vi "Serial_Check.vi"() -> ()   [LabVIEW 2014]
uses:
  <vilib>/Instr/_visa.llb/VISA Configure Serial Port (Instr).vi
  user32.dll
panel:
  in  "정지":bool
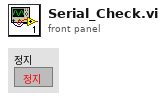
[diagram p1: front panel]
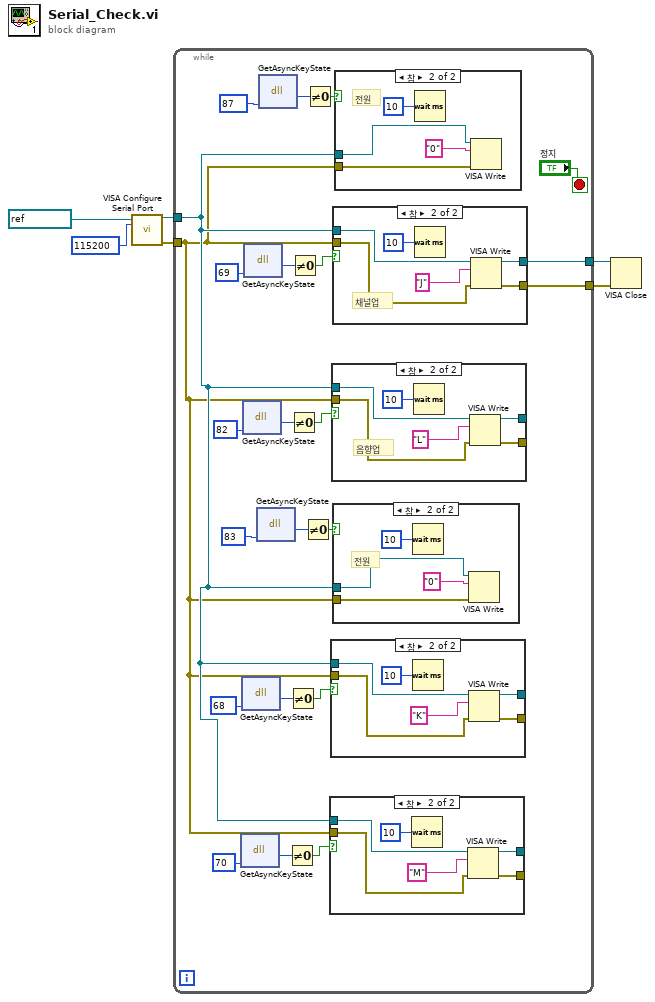
[diagram p0: block diagram]
diagram:
  n1 = call-poly "VISA Configure Serial Port"("VISA resource name"=refnum<visa-resource-name> "COM3", "baud rate (9600)"=u32 115200) -> ("VISA resource name out"=w4:refnum<visa-resource-name>, "error out"=w5:errorcluster)  [unwired: 12 in]
  n2 = while {
    tunnel: w5 -> [w7]
    tunnel: w4 -> [w8]
    tunnel: [w28] -> w3
    tunnel: [w27] -> w2
    stop <- "정지" stop-if-true
    n3 = dll-call lib="User32.dll" fn="GetAsyncKeyState"("vKey"=u8 70 ("Receive_Interaction")) -> ("return type"=w17:i64)  [unwired: 4 in, 2 out]
    n4 = dll-call lib="User32.dll" fn="GetAsyncKeyState"("vKey"=u8 68 ("Receive_Interaction")) -> ("return type"=w12:i64)  [unwired: 4 in, 2 out]
    n5 = dll-call lib="User32.dll" fn="GetAsyncKeyState"("vKey"=u8 82 ("Receive_Interaction")) -> ("return type"=w18:i64)  [unwired: 4 in, 2 out]
    n6 = dll-call lib="User32.dll" fn="GetAsyncKeyState"("vKey"=u8 69 ("Receive_Interaction")) -> ("return type"=w23:i64)  [unwired: 4 in, 2 out]
    n7 = dll-call lib="User32.dll" fn="GetAsyncKeyState"("vKey"=u8 83 ("Receive_Interaction")) -> ("return type"=w10:i64)  [unwired: 4 in, 2 out]
    n8 = dll-call lib="User32.dll" fn="GetAsyncKeyState"("vKey"=u8 87 ("Receive_Interaction")) -> ("return type"=w25:i64)  [unwired: 4 in, 2 out]
    n9 = Not Equal To 0?(x=w17) -> (x != 0?=w15:bool)
    n10 = Not Equal To 0?(x=w12) -> (x != 0?=w14:bool)
    n11 = Not Equal To 0?(x=w18) -> (x != 0?=w20:bool)
    n12 = Not Equal To 0?(x=w23) -> (x != 0?=w21:bool)
    n13 = Not Equal To 0?(x=w10) -> (x != 0?=w11:bool)
    n14 = Not Equal To 0?(x=w25) -> (x != 0?=w24:bool)
    n15 = case shown="참" w15 {
      tunnel: w7 -> [w30 w36]
      tunnel: w8 -> [w31 w35]
      tunnel: [w31 w34] -> _
      tunnel: [w30 w33] -> _
      frame False {
      }
      frame True {
        n16 = Wait (ms)(milliseconds to wait=u32 10 ("대기 시간(ms)")) -> ()  [unwired: 1 out]
        n17 = VISA Write(VISA resource name=w35, write buffer="M", error in (no error)=w36) -> (VISA resource name out=w34:refnum<visa-resource-name>, error out=w33:errorcluster)  [unwired: 1 out]
      }
    }
    n18 = case shown="참" w14 {
      tunnel: w7 -> [w42 w48]
      tunnel: w8 -> [w43 w47]
      tunnel: [w43 w46] -> _
      tunnel: [w42 w45] -> _
      frame False {
      }
      frame True {
        n19 = Wait (ms)(milliseconds to wait=u32 10 ("대기 시간(ms)")) -> ()  [unwired: 1 out]
        n20 = VISA Write(VISA resource name=w47, write buffer="K", error in (no error)=w48) -> (VISA resource name out=w46:refnum<visa-resource-name>, error out=w45:errorcluster)  [unwired: 1 out]
      }
    }
    n21 = case shown="참" w20 {
      tunnel: w7 -> [w50 w56]
      tunnel: w8 -> [w51 w55]
      tunnel: [w51 w54] -> _
      tunnel: [w50 w53] -> _
      frame False {
      }
      frame True {
        # "음향업"
        n22 = Wait (ms)(milliseconds to wait=u32 10 ("대기 시간(ms)")) -> ()  [unwired: 1 out]
        n23 = VISA Write(VISA resource name=w55, write buffer="L", error in (no error)=w56) -> (VISA resource name out=w54:refnum<visa-resource-name>, error out=w53:errorcluster)  [unwired: 1 out]
      }
    }
    n24 = case shown="참" w21 {
      tunnel: w7 -> [w62 w68]
      tunnel: w8 -> [w63 w67]
      tunnel: [w63 w66] -> w28
      tunnel: [w62 w65] -> w27
      frame False {
      }
      frame True {
        # "채널업"
        n25 = Wait (ms)(milliseconds to wait=u32 10 ("대기 시간(ms)")) -> ()  [unwired: 1 out]
        n26 = VISA Write(VISA resource name=w67, write buffer="J", error in (no error)=w68) -> (VISA resource name out=w66:refnum<visa-resource-name>, error out=w65:errorcluster)  [unwired: 1 out]
      }
    }
    n27 = case shown="참" w11 {
      tunnel: w7 -> [_ w40]
      tunnel: w8 -> [_ w39]
      frame False {
      }
      frame True {
        # "전원"
        n28 = Wait (ms)(milliseconds to wait=u32 10 ("대기 시간(ms)")) -> ()  [unwired: 1 out]
        n29 = VISA Write(VISA resource name=w39, write buffer="0" ("write buffer 2"), error in (no error)=w40) -> ()  [unwired: 3 out]
      }
    }
    n30 = case shown="참" w24 {
      tunnel: w7 -> [_ w60]
      tunnel: w8 -> [_ w59]
      frame False {
      }
      frame True {
        # "전원"
        n31 = Wait (ms)(milliseconds to wait=u32 10 ("대기 시간(ms)")) -> ()  [unwired: 1 out]
        n32 = VISA Write(VISA resource name=w59, write buffer="0" ("write buffer 2"), error in (no error)=w60) -> ()  [unwired: 3 out]
      }
    }
  }
  n33 = VISA Close(VISA resource name=w3, error in (no error)=w2) -> ()  [unwired: 1 out]
